vi "Assert.vi"(4 "Variable Y":variant, 6 "Variable X":variant, 11 "Assert Equal in":refnum<class "Assert Greater.lvclass">) -> (2 "Assert?":bool)   [LabVIEW 2019, in "Run Time Assertions.lvlib" / "Assert Greater.lvclass"]
uses:
  <vilib>/gpm_packages/@cs/run-time-assertions/Source/Assert Greater/Assert Greater.lvclass
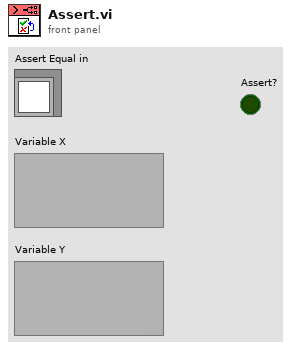
[diagram p1: front panel]
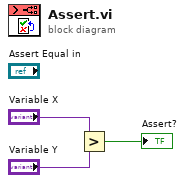
[diagram p0: block diagram]
diagram:
  n1 = Greater?(x="Variable X", y="Variable Y") -> (0:→"Assert?":bool)
